vi "autoDrive.vi"(4 "Distance":dbl) -> (0 "right speed":dbl, 1 "left speed":dbl, 2 "finished?":bool)   [LabVIEW 2013]
doc: "Will drive the robot at a specified speed for a specified distance. Pretty simple."
uses:
  typedefs/State Machine/subStates.ctl
  <vilib>/addons/control/pid/pid.llb/PID (DBL).vi
  <vilib>/addons/control/pid/NI_PID_pid.lvlib
panel:
  out "right desired rate":dbl
  out "left desired rate":dbl
  out "leftDistance":dbl
  out "rightDistance":dbl
  out "leftRate":dbl
  out "rightRate":dbl
  # "Encoder Data"
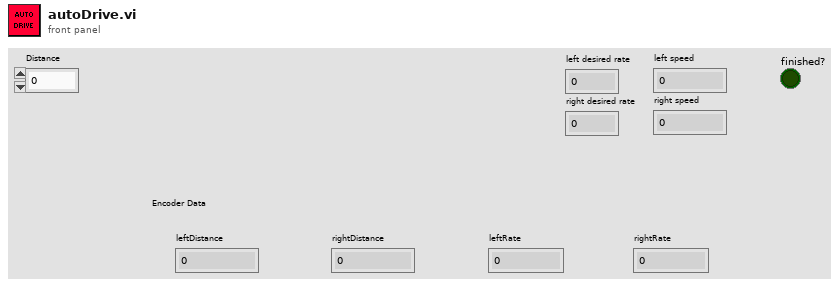
[diagram p1: front panel]
types:
  T1 = cluster{"proportional gain (Kc)":dbl, "integral time (Ti, min)":dbl, "derivative time (Td, min)":dbl}
  T2 = typedef "subStates.ctl" = enum16{"null", "wait", "driver control", "auto", "manual override", "hold position", "rotate", "test", "end"}
  T3 = typedef "WPI_EncoderDevRef.ctl" = cluster{"DevStatus":errorcluster, "EncoderIndex":T4, "CounterIndex":T5, "DistancePerCount":dbl, "Decoding Type":T6}
  T4 = typedef "FPGA_EncoderIdx.ctl" = enum8{"Enc 0", "Enc 1", "Enc 2", "Enc 3", "Invalid"}
  T5 = typedef "FPGA_CounterCtrSystemIndex.ctl" = enum8{"Ctr 0", "Ctr 1", "Ctr 2", "Ctr 3", "Ctr 4", "Ctr 5", "Ctr 6", "Ctr 7", "Invalid"}
  T6 = typedef "WPI_EncoderType.ctl" = enum16{"1x", "2x", "4x"}
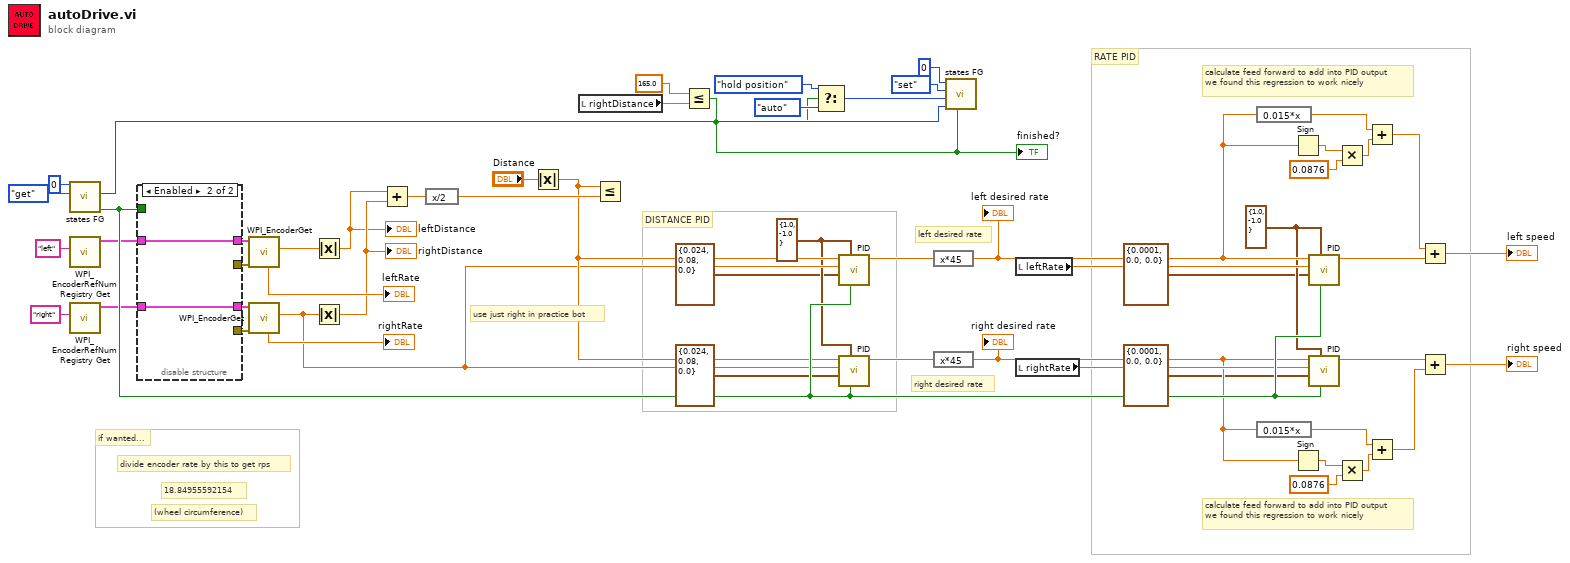
[diagram p0: block diagram]
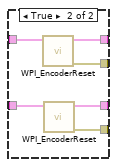
[diagram p3: hidden frame]
diagram:
  w12 = cluster{"output high":dbl, "output low":dbl} {"output high"=1.0, "output low"=-1.0} ("output range")
  w21 = cluster{"output high":dbl, "output low":dbl} {"output high"=1.0, "output low"=-1.0} ("output range")
  # "if wanted..."
  # "RATE PID"
  # "calculate feed forward to add into PID output\nwe found this regression to work nicely"
  # "calculate feed forward to add into PID output\nwe found this regression to work nicely"
  # "DISTANCE PID"
  # "left desired rate"
  # "right desired rate"
  # "use just right in practice bot"
  # "(wheel circumference)"
  # "divide encoder rate by this to get rps"
  # "18.84955592154"
  n1 = call "states FG.vi"("menu (get)"=enum16{"set", "get"}."get", "Loop ID"=0) -> ("first call?"=w56:bool, "state # out"=w48:i32)  [unwired: 6 in, 2 out]
  n2 = call <vilib>:"WPI_EncoderRefNum Registry Get.vi"("refnum name"="left") -> ("EncoderDevRef"=w27:T3)  [unwired: 9 in, 1 out]
  n3 = call <vilib>:"WPI_EncoderRefNum Registry Get.vi"("refnum name"="right") -> ("EncoderDevRef"=w26:T3)  [unwired: 9 in, 1 out]
  n4 = disable-structure shown="Enabled" {
    disable-tunnel: w27 -> [w63 w73]
    disable-tunnel: w26 -> [w62 w72]
    disable-tunnel: [w61 _] -> w54
    disable-tunnel: [w60 w73] -> w53
    disable-tunnel: [w59 w72] -> w52
    disable-tunnel: [w58 _] -> w51
    disable-tunnel: w56 -> [w57 _]
    frame Disabled {
      n5 = case shown="False" w57 {
        tunnel: w63 -> [w65 w70]
        tunnel: w62 -> [w64 w68]
        tunnel: [_ w71] -> w61
        tunnel: [w65 w69] -> w60
        tunnel: [w64 w67] -> w59
        tunnel: [_ w66] -> w58
        frame False {
        }
        frame True {
          n6 = call <vilib>:"WPI_EncoderReset.vi"("EncoderDevRef"=w70) -> ("error out"=w71:errorcluster, "EncoderDevRef"=w69:T3)  [unwired: 9 in]
          n7 = call <vilib>:"WPI_EncoderReset.vi"("EncoderDevRef"=w68) -> ("error out"=w66:errorcluster, "EncoderDevRef"=w67:T3)  [unwired: 9 in]
        }
      }
    }
    frame Enabled {
    }
  }
  n8 = call <vilib>:"WPI_EncoderGet.vi"("error in (no error)"=w54, "EncoderDevRef"=w53) -> ("Distance"=w29:dbl, "Rate"=→"leftRate":dbl)  [unwired: 4 in, 4 out]
  n9 = call <vilib>:"WPI_EncoderGet.vi"("error in (no error)"=w51, "EncoderDevRef"=w52) -> ("Distance"=w28:dbl, "Rate"=→"rightRate":dbl)  [unwired: 4 in, 4 out]
  n10 = Absolute Value(x=w29) -> (abs(x)=w36:dbl)
  "leftDistance" <- w36
  n11 = Absolute Value(x=w28) -> (abs(x)=w39:dbl)
  "rightDistance" <- w39
  n12 = Add(x=w36, y=w39) -> (x+y=w38:dbl)
  n13 = expression code="x/2"(w38) -> (w37:dbl)
  n14 = Absolute Value(x="Distance") -> (abs(x)=w32:dbl)
  n15 = local read "rightDistance"() -> (w33:dbl)
  n16 = Less Or Equal?(x=w32, y=w37) -> ()  [unwired: 1 out]
  n17 = Less Or Equal?(x=165.0, y=w33) -> (x <= y?=w16:bool)
  "finished?" <- w16
  n18 = Select(t=subStates."hold position" ("subState in"), s=w16, f=subStates."auto") -> (s? t:f=w34:T2)
  n19 = call-poly <vilib>:"PID.vi"("reinitialize? (F)"=w56, "output range"=w21, "PID gains"=T1 {"proportional gain (Kc)"=0.024, "integral time (Ti, min)"=0.08, "derivative time (Td, min)"=0.0} ("Left Distance PID gains"), "process variable"=w28, "setpoint"=w32) -> ("output"=w23:dbl)  [unwired: 5 in, 1 out]
  n20 = call-poly <vilib>:"PID.vi"("reinitialize? (F)"=w56, "output range"=w21, "PID gains"=T1 {"proportional gain (Kc)"=0.024, "integral time (Ti, min)"=0.08, "derivative time (Td, min)"=0.0} ("Right Distance PID gains"), "process variable"=w28, "setpoint"=w32) -> ("output"=w22:dbl)  [unwired: 5 in, 1 out]
  n21 = expression code="x*45"(w23) -> (w41:dbl)
  "left desired rate" <- w41
  n22 = expression code="x*45"(w22) -> (w40:dbl)
  "right desired rate" <- w40
  n23 = call "states FG.vi"("exit in"=w16, "state # in"=w48, "subState in"=w34, "menu (get)"=enum16{"set", "get"}."set", "Loop ID"=0) -> ()  [unwired: 3 in, 4 out]
  n24 = local read "leftRate"() -> (w43:dbl)
  n25 = local read "rightRate"() -> (w42:dbl)
  n26 = expression code="0.015*x"(w41) -> (w8:dbl)
  n27 = expression code="0.015*x"(w40) -> (w5:dbl)
  n28 = Sign(1:w41) -> (0:w11:dbl)
  n29 = Sign(1:w40) -> (0:w2:dbl)
  n30 = call-poly <vilib>:"PID.vi"("reinitialize? (F)"=w56, "output range"=w12, "PID gains"=T1 {"proportional gain (Kc)"=0.0001, "integral time (Ti, min)"=0.0, "derivative time (Td, min)"=0.0} ("Left Rate PID gains"), "process variable"=w43, "setpoint"=w41) -> ("output"=w7:dbl)  [unwired: 5 in, 1 out]
  n31 = call-poly <vilib>:"PID.vi"("reinitialize? (F)"=w56, "output range"=w12, "PID gains"=T1 {"proportional gain (Kc)"=0.0001, "integral time (Ti, min)"=0.0, "derivative time (Td, min)"=0.0} ("Right Rate PID gains"), "process variable"=w42, "setpoint"=w40) -> ("output"=w13:dbl)  [unwired: 5 in, 1 out]
  n32 = Multiply(x=w11, y=0.0876) -> (x*y=w9:dbl)
  n33 = Multiply(x=w2, y=0.0876) -> (x*y=w4:dbl)
  n34 = Add(x=w8, y=w9) -> (x+y=w6:dbl)
  n35 = Add(x=w5, y=w4) -> (x+y=w15:dbl)
  n36 = Add(x=w6, y=w7) -> (x+y=→"left speed":dbl)
  n37 = Add(x=w13, y=w15) -> (x+y=→"right speed":dbl)
